vi "RW Constant Edge ROI.vi"(7 "Read/Write":enum16{"Read", "Write"}(ring), 8 "error in (no error)":errorcluster, 11 "Inspec part":T1) -> (0 "error out":errorcluster)   [LabVIEW 2017]
uses:
  Use Module/Algorithm Loop/Gentex Algo/inspec part.ctl
  File/Control/Parent path.ctl
  Toolbox/Control/CVT Action.ctl
  Toolbox/Control/CVT name.vi
  Section and key name.vi
  <vilib>/Utility/config.llb/Write Key (I32).vi
  <vilib>/Utility/config.llb/Write Key (Double).vi
  <vilib>/Utility/config.llb/Read Key (I32).vi
  <vilib>/Utility/config.llb/Read Key (Double).vi
  File/File.lvlib
  <vilib>/Utility/config.llb/NI_LVConfig.lvlib
  Toolbox/Toolbox.lvlib
  Use Module/Algorithm Loop/Algorithm API.lvlib
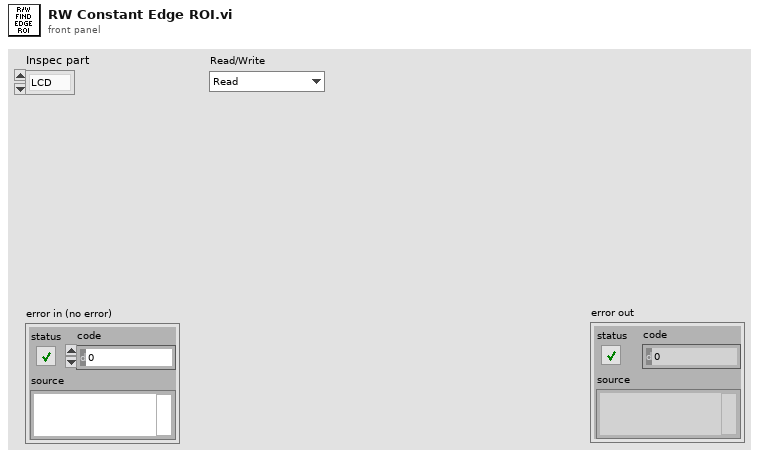
[diagram p1: front panel]
types:
  T1 = typedef "Algorithm API.lvlib/inspec part.ctl" = enum16{"LCD", "Housing"}
  T2 = typedef "File.lvlib/Parent path.ctl" = enum16{"Project", "Setting", "Log"}
  T3 = typedef "Toolbox.lvlib/CVT Action.ctl" = enum16{"Set", "Replace", "Get", "Check", "Delete", "Delete All"}
  T4 = typedef "ROI Descriptor" = cluster{"Global Rectangle":i32[], "Contours":cluster{"ID":enum32{"External", "Internal"}, "Type":u32, "Coordinates":i32[]}[]}
  T5 = typedef "IMAQ Rectangle" = cluster{"Left":i32, "Top":i32, "Right":i32, "Bottom":i32, "Rotation":dbl}
  T6 = typedef "NI_LVConfig.lvlib/Config Data RefNum.ctl" = refnum<k1>
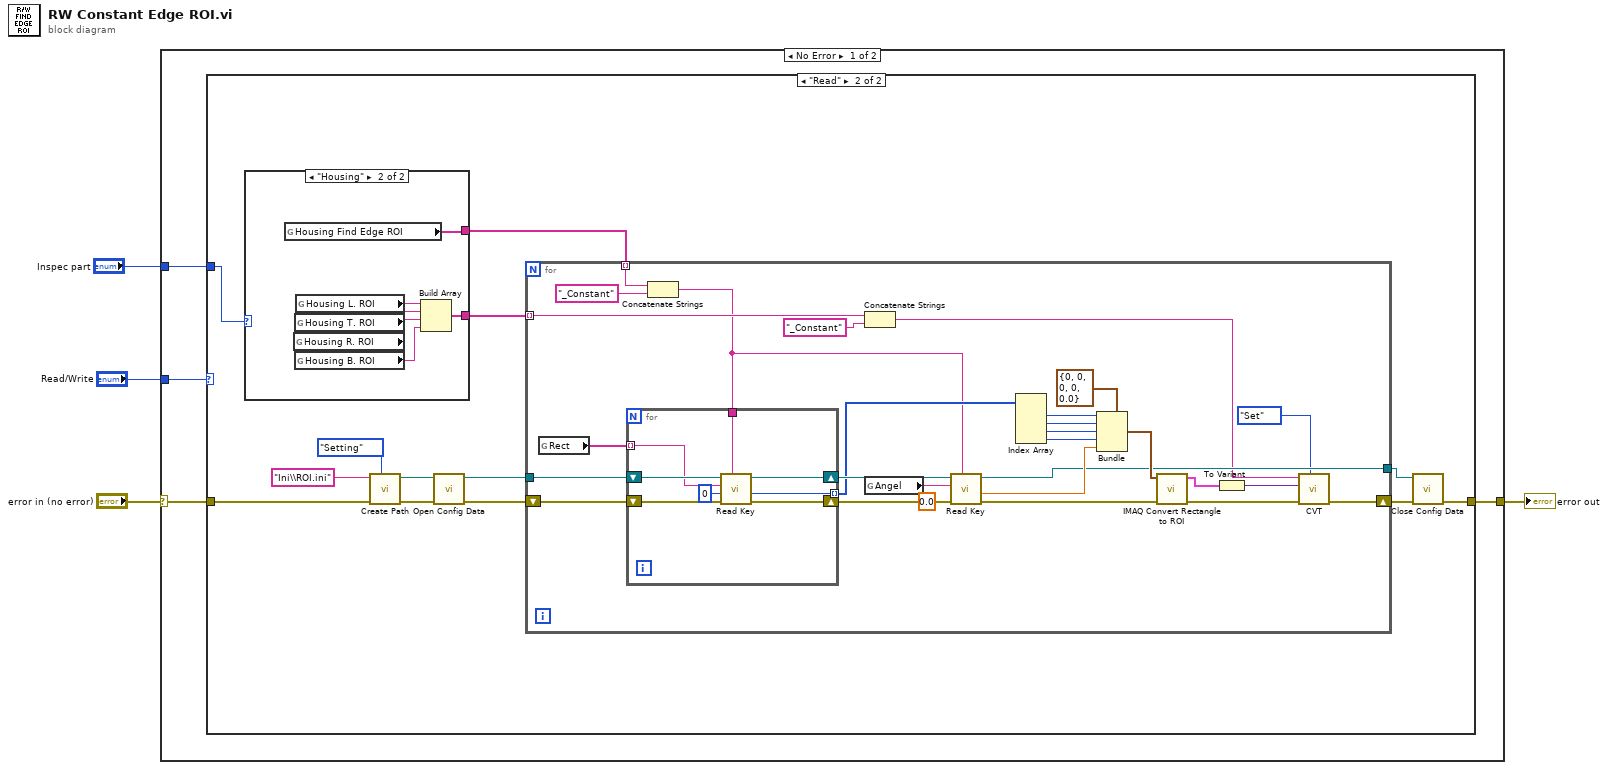
[diagram p0: block diagram]
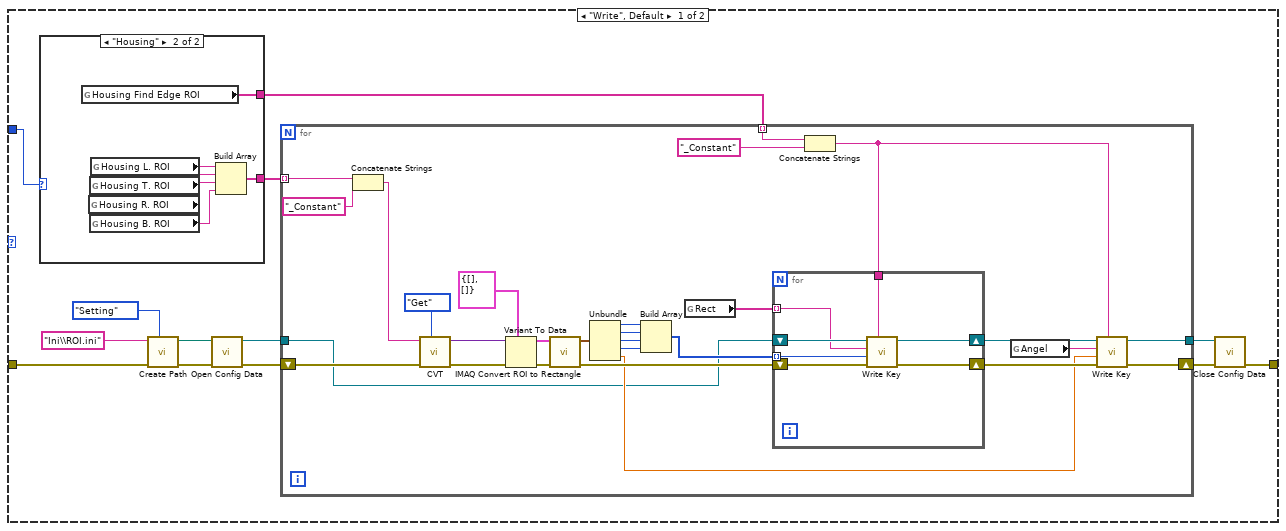
[diagram p2: hidden frame]
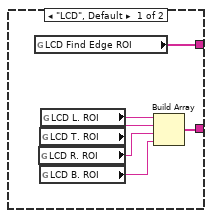
[diagram p3: hidden frame]
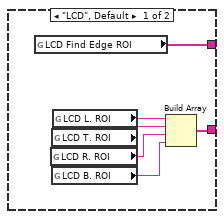
[diagram p4: hidden frame]
diagram:
  n1 = case shown="No Error" "error in (no error)" {
    selector: "error in (no error)" -> [w8 w130]
    tunnel: [w7 w130] -> w3
    tunnel: "Read/Write" -> [w6 _]
    tunnel: "Inspec part" -> [w5 _]
    frame No Error {
      n2 = case shown="\"Read\"" w6 {
        tunnel: w8 -> [w21 w81]
        tunnel: [w14 w74] -> w7
        tunnel: w5 -> [w10 w70]
        frame "Write", Default {
          n3 = case shown="\"Housing\"" w10 {
            tunnel: [w23 w29] -> w11
            tunnel: [w22 w28] -> w9
            frame "LCD", Default {
              n4 = global read "Section and key name.vi" "LCD Find Edge ROI"() -> (w22:string[])
              n5 = global read "CVT name.vi" "LCD R. ROI"() -> (w25:string)
              n6 = global read "CVT name.vi" "LCD T. ROI"() -> (w26:string)
              n7 = global read "CVT name.vi" "LCD B. ROI"() -> (w24:string)
              n8 = global read "CVT name.vi" "LCD L. ROI"() -> (w27:string)
              n9 = Build Array(w27, w26, w25, w24) -> (w23:string[])
            }
            frame "Housing" {
              n10 = global read "Section and key name.vi" "Housing Find Edge ROI"() -> (w28:string[])
              n11 = global read "CVT name.vi" "Housing R. ROI"() -> (w31:string)
              n12 = global read "CVT name.vi" "Housing T. ROI"() -> (w32:string)
              n13 = global read "CVT name.vi" "Housing B. ROI"() -> (w30:string)
              n14 = global read "CVT name.vi" "Housing L. ROI"() -> (w33:string)
              n15 = Build Array(w33, w32, w31, w30) -> (w29:string[])
            }
          }
          n16 = call "Create Path.vi"("Parent path"=Parent_path."Setting", "error in (no error)"=w21, "Directory"="Ini\\ROI.ini") -> ("error out"=w19:errorcluster, "Path"=w18:path)  [unwired: 7 in]
          n17 = call <vilib>:"Open Config Data.vi"("error in (no error)"=w19, "configuration file path"=w18) -> ("error out"=w16:errorcluster, "refnum"=w17:T6)  [unwired: 7 in, 1 out]
          n18 = for {
            tunnel: w17 -> [w39]
            shift-right: [w56] -> w15
            shift-left: w16 -> [w61]
            tunnel: [w55] -> w13
            tunnel: w11 -> [w49] mode=indexing
            tunnel: w9 -> [w38] mode=indexing
            n19 = Concatenate Strings(w49, "_Constant" ("string")) -> (w35:string)
            n20 = call "CVT.vi"("Action"=CVT_Action."Get", "error in (no error)"=w61, "Key"=w35) -> ("error out"=w54:errorcluster, "Value out"=w52:variant)  [unwired: 6 in, 1 out]
            n21 = Variant To Data(error in=w54, type=T4 {"Global Rectangle"=[], "Contours"=[]} ("ROI Descriptor"), Variant=w52) -> (data=w47:T4, error out=w53:errorcluster)
            n22 = call "IMAQ Convert ROI to Rectangle"("error in (no error)"=w53, "ROI Descriptor"=w47) -> ("error out"=w48:errorcluster, "Rectangle"=w46:T5)  [unwired: 7 in]
            n23 = Unbundle(w46) -> ("Left"=w44:i32, "Top"=w43:i32, "Right"=w42:i32, "Bottom"=w41:i32, "Rotation"=w45:dbl)
            n24 = Build Array(w44, w43, w42, w41) -> (w40:i32[])
            n25 = global read "Section and key name.vi" "Rect"() -> (w58:string[])
            n26 = Concatenate Strings(w38, "_Constant" ("string")) -> (w37:string)
            n27 = for {
              shift-right: [w66] -> w60
              shift-left: w39 -> [w68]
              shift-right: [w65] -> w59
              shift-left: w48 -> [w67]
              tunnel: w58 -> [w64] mode=indexing
              tunnel: w37 -> [w63]
              tunnel: w40 -> [w62] mode=indexing
              n28 = call-poly <vilib>:"Write Key.vi"("section"=w63, "error in (no error)"=w67, "value"=w62, "key"=w64, "refnum"=w68) -> ("error out"=w65:errorcluster, "refnum out"=w66:T6)  [unwired: 4 in, 1 out]
            }
            n29 = global read "Section and key name.vi" "Angel"() -> (w57:string)
            n30 = call-poly <vilib>:"Write Key.vi"("section"=w37, "error in (no error)"=w59, "value"=w45, "key"=w57, "refnum"=w60) -> ("error out"=w56:errorcluster, "refnum out"=w55:T6)  [unwired: 4 in, 1 out]
          }
          n31 = call <vilib>:"Close Config Data.vi"("error in (no error)"=w15, "refnum"=w13) -> ("error out"=w14:errorcluster)  [unwired: 8 in, 1 out]
        }
        frame "Read" {
          n32 = case shown="\"Housing\"" w70 {
            tunnel: [w83 w89] -> w72
            tunnel: [w82 w88] -> w69
            frame "LCD", Default {
              n33 = global read "Section and key name.vi" "LCD Find Edge ROI"() -> (w82:string[])
              n34 = global read "CVT name.vi" "LCD R. ROI"() -> (w85:string)
              n35 = global read "CVT name.vi" "LCD T. ROI"() -> (w86:string)
              n36 = global read "CVT name.vi" "LCD B. ROI"() -> (w84:string)
              n37 = global read "CVT name.vi" "LCD L. ROI"() -> (w87:string)
              n38 = Build Array(w87, w86, w85, w84) -> (w83:string[])
            }
            frame "Housing" {
              n39 = global read "Section and key name.vi" "Housing Find Edge ROI"() -> (w88:string[])
              n40 = global read "CVT name.vi" "Housing R. ROI"() -> (w91:string)
              n41 = global read "CVT name.vi" "Housing T. ROI"() -> (w92:string)
              n42 = global read "CVT name.vi" "Housing B. ROI"() -> (w90:string)
              n43 = global read "CVT name.vi" "Housing L. ROI"() -> (w93:string)
              n44 = Build Array(w93, w92, w91, w90) -> (w89:string[])
            }
          }
          n45 = call "Create Path.vi"("Parent path"=Parent_path."Setting", "error in (no error)"=w81, "Directory"="Ini\\ROI.ini") -> ("error out"=w79:errorcluster, "Path"=w78:path)  [unwired: 7 in]
          n46 = call <vilib>:"Open Config Data.vi"("error in (no error)"=w79, "configuration file path"=w78) -> ("error out"=w76:errorcluster, "refnum"=w77:T6)  [unwired: 7 in, 1 out]
          n47 = for {
            tunnel: w77 -> [w121]
            shift-right: [w104] -> w75
            shift-left: w76 -> [w120]
            tunnel: [w105] -> w73
            tunnel: w69 -> [w98] mode=indexing
            tunnel: w72 -> [w100] mode=indexing
            n48 = global read "Section and key name.vi" "Rect"() -> (w117:string[])
            n49 = Concatenate Strings(w98, "_Constant" ("string")) -> (w96:string)
            n50 = for {
              shift-right: [w127] -> w119
              shift-left: w121 -> [w129]
              shift-right: [w126] -> w118
              shift-left: w120 -> [w128]
              tunnel: [w125] -> w114 mode=indexing
              tunnel: w117 -> [w124] mode=indexing
              tunnel: w96 -> [w123]
              n51 = call-poly <vilib>:"Read Key.vi"("section"=w123, "error in (no error)"=w128, "default value"=0, "key"=w124, "refnum"=w129) -> ("error out"=w126:errorcluster, "value"=w125:i32, "refnum out"=w127:T6)  [unwired: 3 in, 1 out]
            }
            n52 = Concatenate Strings(w100, "_Constant" ("string")) -> (w95:string)
            n53 = global read "Section and key name.vi" "Angel"() -> (w116:string)
            n54 = call-poly <vilib>:"Read Key.vi"("section"=w96, "error in (no error)"=w118, "default value"=0.0, "key"=w116, "refnum"=w119) -> ("error out"=w115:errorcluster, "value"=w108:dbl, "refnum out"=w105:T6)  [unwired: 3 in, 1 out]
            n55 = Index Array(array=w114) -> (element #1=w112:i32, element #2=w111:i32, element #3=w110:i32, element #4=w109:i32)  [unwired: 4 in]
            n56 = Bundle(cluster=T5 {"Left"=0, "Top"=0, "Right"=0, "Bottom"=0, "Rotation"=0.0} ("Rectangle"), "Left"=w112, "Top"=w111, "Right"=w110, "Bottom"=w109, "Rotation"=w108) -> (w107:T5)
            n57 = call "IMAQ Convert Rectangle to ROI"("error in (no error)"=w115, "Rectangle"=w107) -> ("error out"=w106:errorcluster, "ROI Descriptor"=w103:T4)  [unwired: 7 in]
            n58 = To Variant(anything=w103) -> (Variant=w102:variant)
            n59 = call "CVT.vi"("Action"=CVT_Action."Set", "error in (no error)"=w106, "Value in"=w102, "Key"=w95) -> ("error out"=w104:errorcluster)  [unwired: 5 in, 2 out]
          }
          n60 = call <vilib>:"Close Config Data.vi"("error in (no error)"=w75, "refnum"=w73) -> ("error out"=w74:errorcluster)  [unwired: 8 in, 1 out]
        }
      }
    }
    frame Error {
    }
  }
  "error out" <- w3
